vi "Proximity sensor display.vi"(8 "Right Ultrasonic Value":dbl, 9 "Left Ultrasonic Value":dbl, 10 "Back Ultrasonic Value":dbl, 11 "Front Ultrasonic Value":dbl) -> ()   [LabVIEW 2016]
uses:
  <vilib>/Rock Robotics/Network Tables/NT Write Boolean.vi
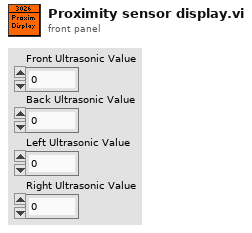
[diagram p1: front panel]
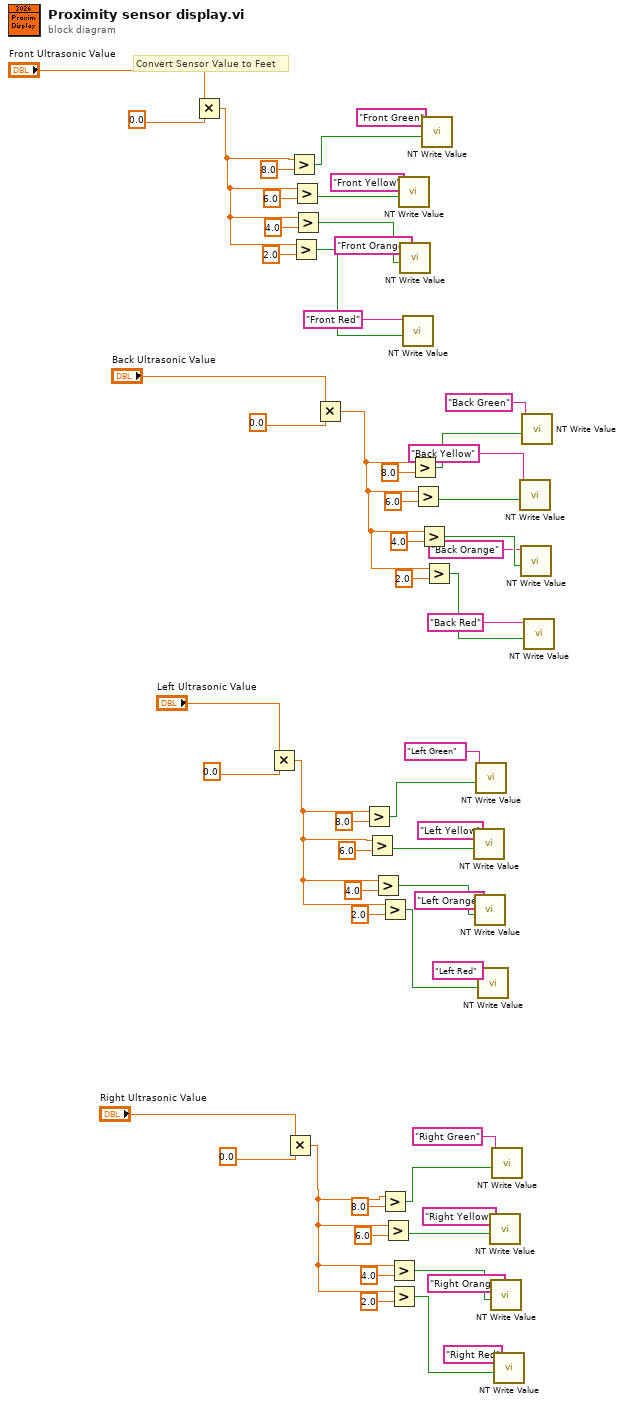
[diagram p0: block diagram]
diagram:
  # "Convert Sensor Value to Feet"
  n1 = Multiply(x="Front Ultrasonic Value", y=0.0) -> (x*y=w17:dbl)
  n2 = Multiply(x="Left Ultrasonic Value", y=0.0) -> (x*y=w19:dbl)
  n3 = Multiply(x="Right Ultrasonic Value", y=0.0) -> (x*y=w18:dbl)
  n4 = Greater?(x=w17, y=8.0) -> (0:w58:bool)
  n5 = Greater?(x=w17, y=2.0) -> (0:w55:bool)
  n6 = Greater?(x=w17, y=6.0) -> (0:w57:bool)
  n7 = Greater?(x=w17, y=4.0) -> (0:w56:bool)
  n8 = Multiply(x="Back Ultrasonic Value", y=0.0) -> (x*y=w20:dbl)
  n9 = Greater?(x=w19, y=8.0) -> (0:w39:bool)
  n10 = Greater?(x=w19, y=6.0) -> (0:w38:bool)
  n11 = Greater?(x=w19, y=4.0) -> (0:w37:bool)
  n12 = Greater?(x=w19, y=2.0) -> (0:w36:bool)
  n13 = Greater?(x=w18, y=8.0) -> (0:w29:bool)
  n14 = Greater?(x=w18, y=6.0) -> (0:w28:bool)
  n15 = Greater?(x=w18, y=4.0) -> (0:w27:bool)
  n16 = Greater?(x=w18, y=2.0) -> (0:w26:bool)
  n17 = call-poly <vilib>:"NT Write Value.vi"("Boolean"=w57, "Name"="Front Yellow") -> ()  [unwired: 9 in, 1 out]
  n18 = call-poly <vilib>:"NT Write Value.vi"("Boolean"=w56, "Name"="Front Orange") -> ()  [unwired: 9 in, 1 out]
  n19 = call-poly <vilib>:"NT Write Value.vi"("Boolean"=w55, "Name"="Front Red") -> ()  [unwired: 9 in, 1 out]
  n20 = Greater?(x=w20, y=8.0) -> (0:w49:bool)
  n21 = Greater?(x=w20, y=6.0) -> (0:w48:bool)
  n22 = Greater?(x=w20, y=4.0) -> (0:w47:bool)
  n23 = call-poly <vilib>:"NT Write Value.vi"("Boolean"=w58, "Name"="Front Green") -> ()  [unwired: 9 in, 1 out]
  n24 = Greater?(x=w20, y=2.0) -> (0:w46:bool)
  n25 = call-poly <vilib>:"NT Write Value.vi"("Boolean"=w38, "Name"="Left Yellow") -> ()  [unwired: 9 in, 1 out]
  n26 = call-poly <vilib>:"NT Write Value.vi"("Boolean"=w37, "Name"="Left Orange") -> ()  [unwired: 9 in, 1 out]
  n27 = call-poly <vilib>:"NT Write Value.vi"("Boolean"=w39, "Name"="Left Green") -> ()  [unwired: 9 in, 1 out]
  n28 = call-poly <vilib>:"NT Write Value.vi"("Boolean"=w36, "Name"="Left Red") -> ()  [unwired: 9 in, 1 out]
  n29 = call-poly <vilib>:"NT Write Value.vi"("Boolean"=w28, "Name"="Right Yellow") -> ()  [unwired: 9 in, 1 out]
  n30 = call-poly <vilib>:"NT Write Value.vi"("Boolean"=w27, "Name"="Right Orange") -> ()  [unwired: 9 in, 1 out]
  n31 = call-poly <vilib>:"NT Write Value.vi"("Boolean"=w29, "Name"="Right Green") -> ()  [unwired: 9 in, 1 out]
  n32 = call-poly <vilib>:"NT Write Value.vi"("Boolean"=w26, "Name"="Right Red") -> ()  [unwired: 9 in, 1 out]
  n33 = call-poly <vilib>:"NT Write Value.vi"("Boolean"=w48, "Name"="Back Yellow") -> ()  [unwired: 9 in, 1 out]
  n34 = call-poly <vilib>:"NT Write Value.vi"("Boolean"=w47, "Name"="Back Orange") -> ()  [unwired: 9 in, 1 out]
  n35 = call-poly <vilib>:"NT Write Value.vi"("Boolean"=w49, "Name"="Back Green") -> ()  [unwired: 9 in, 1 out]
  n36 = call-poly <vilib>:"NT Write Value.vi"("Boolean"=w46, "Name"="Back Red") -> ()  [unwired: 9 in, 1 out]
